vi "projekt2.vi"() -> ()   [LabVIEW 2020]
panel:
  in  "?":bool
  in  "stop":bool
  out "dbl":dbl format="%#.4g"
  in  "Model [0-1]":u8 max=2 step=1
  in  "Rezystancja [DBL]":dbl format="%#.6g"
  in  "Jednostka [0-2]":u8 max=2 step=1
  # "Czujnik"
  # "PT100"
  # "KTY81-210"
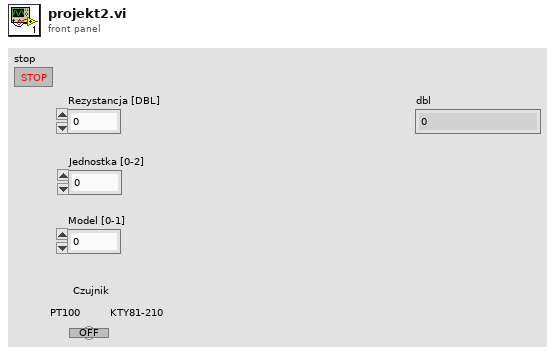
[diagram p1: front panel]
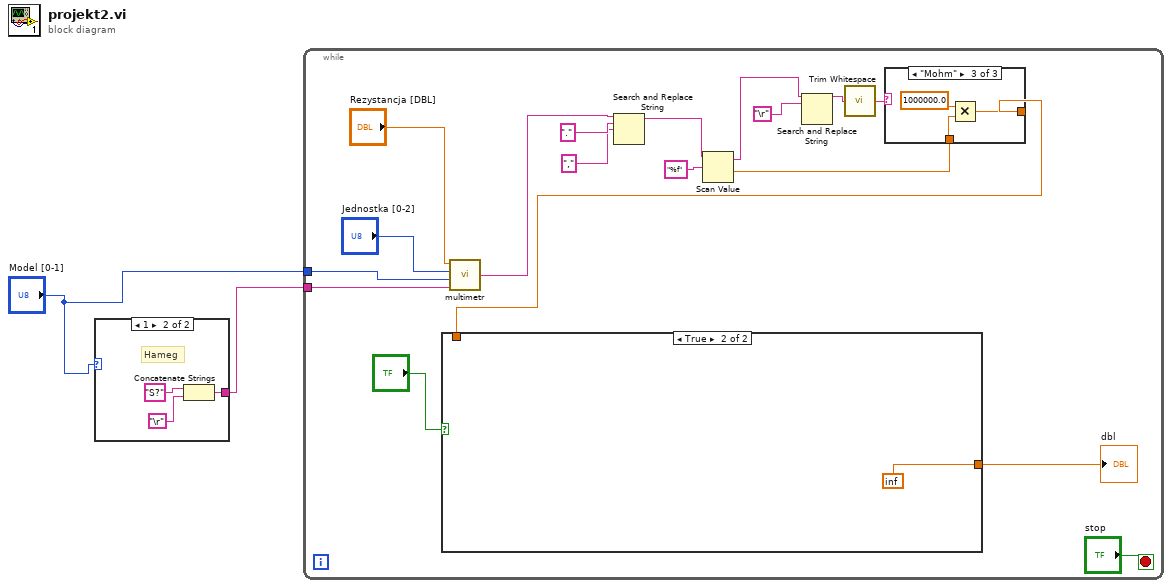
[diagram p0: block diagram]
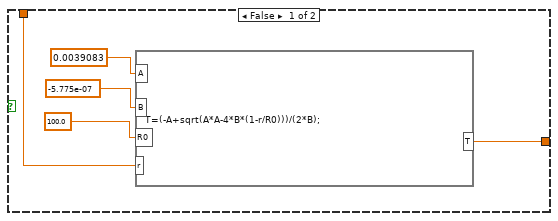
[diagram p2: hidden frame]
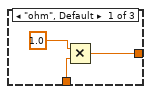
[diagram p3: hidden frame]
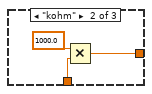
[diagram p4: hidden frame]
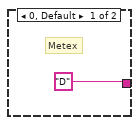
[diagram p5: hidden frame]
diagram:
  n1 = case shown="1" "Model [0-1]" {
    tunnel: ["D" w4] -> w1
    frame 0, Default {
      # "Metex"
    }
    frame 1 {
      # "Hameg"
      n2 = Concatenate Strings("S?", "\r") -> (w4:string)
    }
  }
  n3 = while {
    tunnel: "Model [0-1]" -> [w24]
    tunnel: w1 -> [w23]
    stop <- "stop" stop-if-true
    n4 = call "multimetr.vi"("Zapytanie"=w23, "Model [0-1]"=w24, "Jednostka [0-2]"="Jednostka [0-2]", "Rezystancja [DBL]"="Rezystancja [DBL]") -> ("Ramka"=w19:string)
    n5 = Search and Replace String(input string=w19, search string=".", replace string=",") -> (result string=w20:string)  [unwired: 5 in, 3 out]
    n6 = Scan Value(string=w20, format string="%f") -> (output string=w14:string, value=w15:dbl)  [unwired: 1 in]
    n7 = Search and Replace String(input string=w14, search string="\r") -> (result string=w11:string)  [unwired: 6 in, 3 out]
    n8 = call <vilib>:"Trim Whitespace.vi"("string"=w11) -> ("trimmed string"=w10:string)  [unwired: 1 in]
    n9 = case shown="\"Mohm\"" w10 {
      tunnel: w15 -> [w32 w35 w38]
      tunnel: [w31 w34 w37] -> w8
      frame "ohm", Default {
        n10 = Multiply(x=1.0, y=w32) -> (x*y=w31:dbl)
      }
      frame "kohm" {
        n11 = Multiply(x=1000.0, y=w35) -> (x*y=w34:dbl)
      }
      frame "Mohm" {
        n12 = Multiply(x=1000000.0, y=w38) -> (x*y=w37:dbl)
      }
    }
    n13 = case shown="True" "?" {
      tunnel: w8 -> [w26 _]
      tunnel: [w25 inf] -> w7
      frame False {
        n14 = formula code="T=(-A+sqrt(A*A-4*B*(1-r/R0)))/(2*B);"("A"=0.0039083, "B"=-5.775e-07, "R0"=100.0, "r"=w26) -> ("T"=w25:dbl)
      }
      frame True {
      }
    }
    "dbl" <- w7
  }
